vi "CVT MUS2MIDI controller.vi"(8 "error in":errorcluster, 11 "MSU set":u8) -> (0 "error out":errorcluster, 3 "midi_ctrl":u8)   [LabVIEW 8.6]
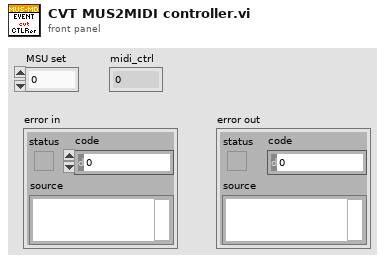
[diagram p1: front panel]
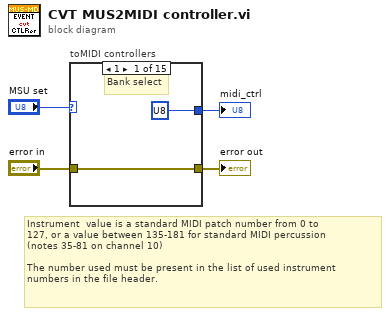
[diagram p0: block diagram]
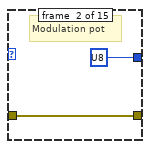
[diagram p2: hidden frame]
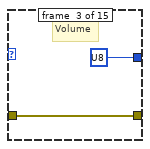
[diagram p3: hidden frame]
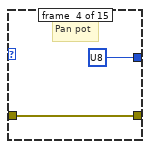
[diagram p4: hidden frame]
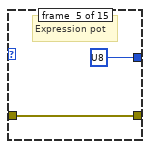
[diagram p5: hidden frame]
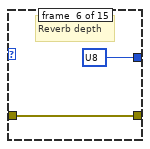
[diagram p6: hidden frame]
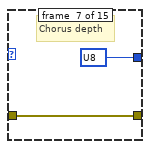
[diagram p7: hidden frame]
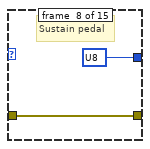
[diagram p8: hidden frame]
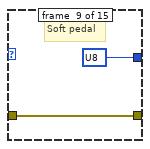
[diagram p9: hidden frame]
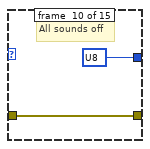
[diagram p10: hidden frame]
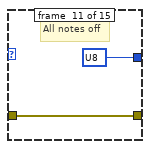
[diagram p11: hidden frame]
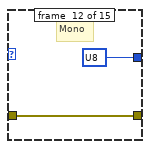
[diagram p12: hidden frame]
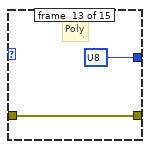
[diagram p13: hidden frame]
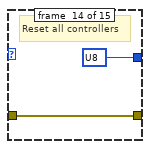
[diagram p14: hidden frame]
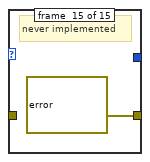
[diagram p15: hidden frame]
diagram:
  # "Instrument  value is a standard MIDI patch number from 0 to \n127, or a value between 135-181 for standard MIDI percussion \n(notes 35-81 on channel 10)\n\nThe number used must be present in the list of used instrument \nnumbers in the file header."
  n1 = case "toMIDI controllers" shown="1" "MSU set" {
    tunnel: [u8 ? ("data") u8 ? ("data") u8 ? ("data") u8 ? ("data") u8 ? ("data") u8 ? ("data") u8 ? ("data") u8 ? ("data") u8 ? ("data") u8 ? ("data") u8 ? ("data") u8 ? ("data") u8 ? ("data") u8 ? ("data") _] -> w2
    tunnel: [w5 w7 w9 w11 w13 w15 w17 w19 w21 w23 w25 w27 w29 w31 errorcluster ? ("error constant")] -> w4
    tunnel: "error in" -> [w5 w7 w9 w11 w13 w15 w17 w19 w21 w23 w25 w27 w29 w31 _]
    frame #0 {
      # "Bank select"
    }
    frame #1 {
      # "Modulation pot"
    }
    frame #2 {
      # "Volume"
    }
    frame #3 {
      # "Pan pot"
    }
    frame #4 {
      # "Expression pot"
    }
    frame #5 {
      # "Reverb depth"
    }
    frame #6 {
      # "Chorus depth"
    }
    frame #7 {
      # "Sustain pedal"
    }
    frame #8 {
      # "Soft pedal"
    }
    frame #9 {
      # "All sounds off"
    }
    frame #10 {
      # "All notes off"
    }
    frame #11 {
      # "Mono"
    }
    frame #12 {
      # "Poly"
    }
    frame #13 {
      # "Reset all controllers"
    }
    frame #14 {
      # "never implemented"
    }
  }
  "error out" <- w4
  "midi_ctrl" <- w2
